vi "EDITORS_calculate_next_pos_for_keyboard_events.vi"(7 "direction":T1, 9 "SQL_rows":i32, 10 "editable_columns":i32[](array[numeric]), 11 "reference":refnum<vi>) -> ()   [LabVIEW 2019]
uses:
  _misc/directions.ctl
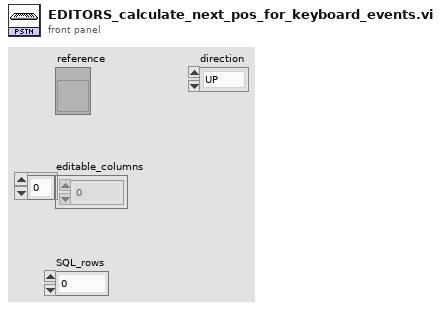
[diagram p1: front panel]
types:
  T1 = typedef "directions.ctl" = enum16{"UP", "DOWN", "LEFT", "RIGHT"}
  T2 = typedef "LVRowAndColumnTypeDef.ctl" = cluster{"Row":i32, "Column":i32}
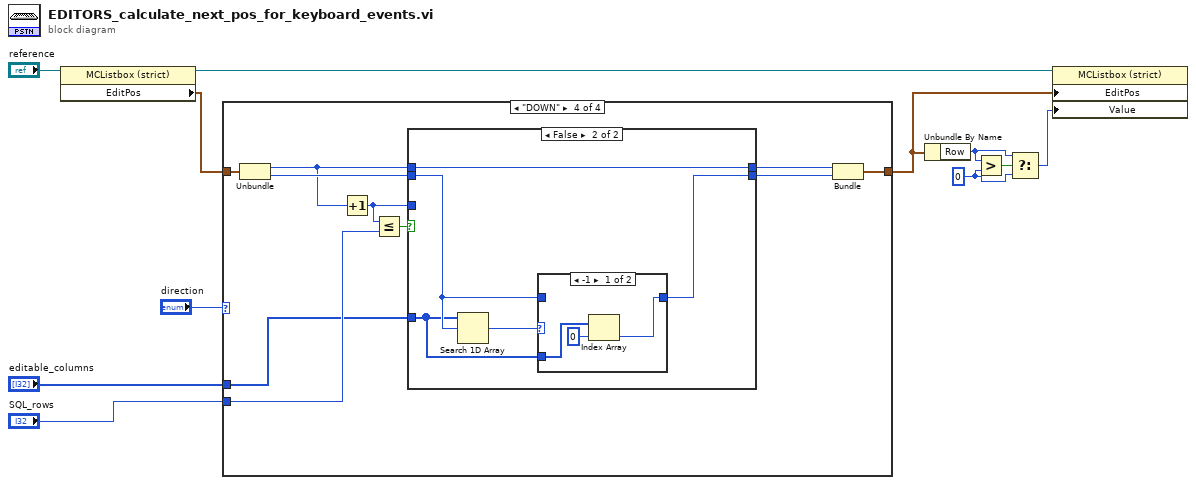
[diagram p0: block diagram]
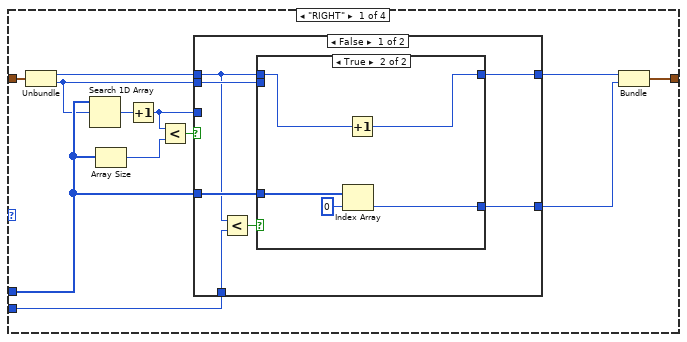
[diagram p2: hidden frame]
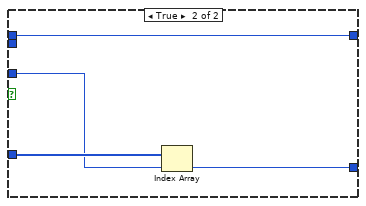
[diagram p4: hidden frame]
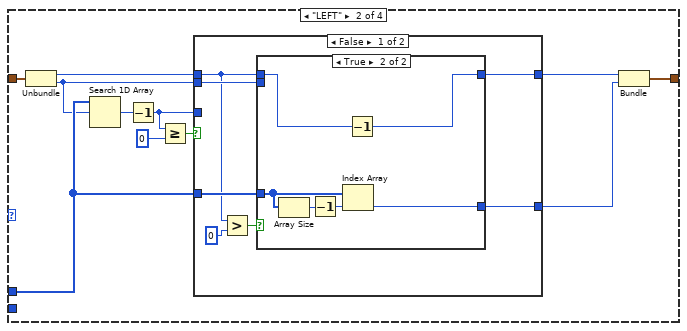
[diagram p5: hidden frame]
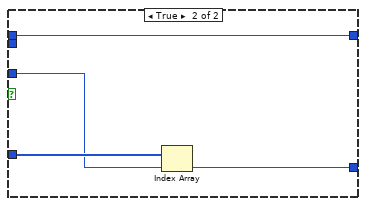
[diagram p7: hidden frame]
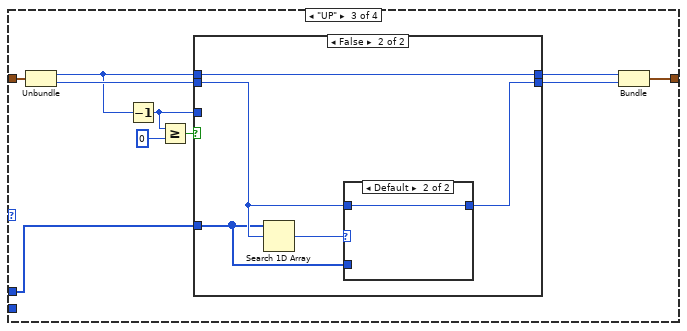
[diagram p8: hidden frame]
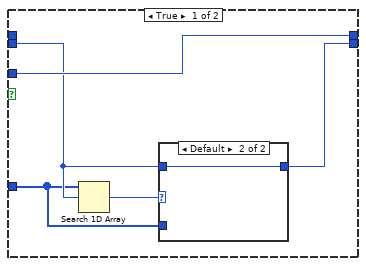
[diagram p9: hidden frame]
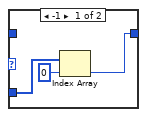
[diagram p10: hidden frame]
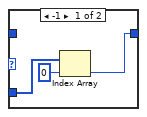
[diagram p11: hidden frame]
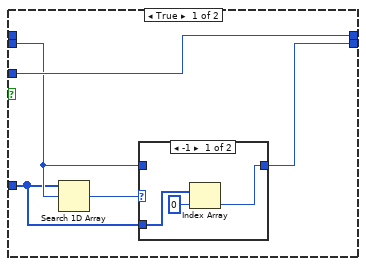
[diagram p12: hidden frame]
diagram:
  w2 = 0 ("lower limit")
  n1 = property on="Property Node" class="MCListbox (strict)"(reference="reference") -> (reference out=w10:refnum<vi>, "EditPos"=w11:T2)  [unwired: 1 in, 1 out]
  n2 = case shown="\"DOWN\"" "direction" {
    tunnel: w11 -> [w23 w52 w81 w109]
    tunnel: [w22 w51 w80 w108] -> w5
    tunnel: "editable_columns" -> [w18 w48 w72 w100]
    tunnel: "SQL_rows" -> [w12 _ _ w101]
    frame "RIGHT" {
      n3 = Unbundle(w23) -> ("Row"=w15:i32, "Column"=w13:i32)
      n4 = Search 1D Array(1D array=w18, element=w13) -> (index of element=w21:i32)  [unwired: 1 in]
      n5 = Array Size(array=w18) -> (size(s)=w20:i32)
      n6 = Increment(x=w21) -> (x+1=w17:i32)
      n7 = Less?(x=w17, y=w20) -> (x < y?=w19:bool)
      n8 = case shown="False" w19 {
        tunnel: w18 -> [w29 w41]
        tunnel: w17 -> [_ w40]
        tunnel: [w28 w39] -> w16
        tunnel: w15 -> [w25 w38]
        tunnel: [w30 w38] -> w14
        tunnel: w13 -> [w27 _]
        tunnel: w12 -> [w24 _]
        frame False {
          n9 = Less?(x=w25, y=w24) -> (x < y?=w26:bool)
          n10 = case shown="True" w26 {
            tunnel: w25 -> [w32 w37]
            tunnel: [w32 w36] -> w30
            tunnel: w29 -> [_ w34]
            tunnel: [w31 w35] -> w28
            tunnel: w27 -> [w31 _]
            frame False {
            }
            frame True {
              n11 = Index Array(array=w34, index=0) -> (element=w35:i32)
              n12 = Increment(x=w37) -> (x+1=w36:i32)
            }
          }
        }
        frame True {
          n13 = Index Array(array=w41, index=w40) -> (element=w39:i32)
        }
      }
      n14 = Bundle("Row"=w14, "Numeric"=w16) -> (w22:cluster{"Row":i32, "Numeric":i32})  [unwired: 1 in]
    }
    frame "LEFT" {
      n15 = Unbundle(w52) -> ("Row"=w45:i32, "Column"=w43:i32)
      n16 = Search 1D Array(1D array=w48, element=w43) -> (index of element=w50:i32)  [unwired: 1 in]
      n17 = Decrement(x=w50) -> (x-1=w47:i32)
      n18 = Greater Or Equal?(x=w47, y=0) -> (x >= y?=w49:bool)
      n19 = case shown="False" w49 {
        tunnel: w48 -> [w58 w71]
        tunnel: w47 -> [_ w70]
        tunnel: [w57 w69] -> w46
        tunnel: w45 -> [w54 w68]
        tunnel: [w59 w68] -> w44
        tunnel: w43 -> [w56 _]
        frame False {
          n20 = Greater?(x=w54, y=0) -> (0:w55:bool)
          n21 = case shown="True" w55 {
            tunnel: w54 -> [w61 w67]
            tunnel: [w61 w66] -> w59
            tunnel: w58 -> [_ w62]
            tunnel: [w60 w65] -> w57
            tunnel: w56 -> [w60 _]
            frame False {
            }
            frame True {
              n22 = Array Size(array=w62) -> (size(s)=w64:i32)
              n23 = Decrement(x=w64) -> (x-1=w63:i32)
              n24 = Index Array(array=w62, index=w63) -> (element=w65:i32)
              n25 = Decrement(x=w67) -> (x-1=w66:i32)
            }
          }
        }
        frame True {
          n26 = Index Array(array=w71, index=w70) -> (element=w69:i32)
        }
      }
      n27 = Bundle("Row"=w44, "Numeric"=w46) -> (w51:cluster{"Row":i32, "Numeric":i32})  [unwired: 1 in]
    }
    frame "UP" {
      n28 = Unbundle(w81) -> ("Row"=w74:i32, "Column"=w76:i32)
      n29 = Decrement(x=w74) -> (x-1=w78:i32)
      n30 = Greater Or Equal?(x=w78, y=0) -> (x >= y?=w79:bool)
      n31 = case shown="False" w79 {
        tunnel: w78 -> [w86 _]
        tunnel: w74 -> [_ w91]
        tunnel: [w86 w91] -> w77
        tunnel: w76 -> [w84 w94]
        tunnel: [w82 w92] -> w73
        tunnel: w72 -> [w83 w93]
        frame True {
          n32 = Search 1D Array(1D array=w83, element=w84) -> (index of element=w85:i32)  [unwired: 1 in]
          n33 = case shown="Default" w85 {
            tunnel: w84 -> [_ w90]
            tunnel: [w87 w90] -> w82
            tunnel: w83 -> [w89 _]
            frame -1 {
              n34 = Index Array(array=w89, index=0) -> (element=w87:i32)
            }
            frame Default {
            }
          }
        }
        frame False {
          n35 = Search 1D Array(1D array=w93, element=w94) -> (index of element=w95:i32)  [unwired: 1 in]
          n36 = case shown="Default" w95 {
            tunnel: w94 -> [_ w99]
            tunnel: [w96 w99] -> w92
            tunnel: w93 -> [w98 _]
            frame -1 {
              n37 = Index Array(array=w98, index=0) -> (element=w96:i32)
            }
            frame Default {
            }
          }
        }
      }
      n38 = Bundle("Row"=w77, "Column"=w73) -> (w80:cluster{"Row":i32, "Column":i32})  [unwired: 1 in]
    }
    frame "DOWN" {
      n39 = Unbundle(w109) -> ("Row"=w103:i32, "Column"=w104:i32)
      n40 = Increment(x=w103) -> (x+1=w106:i32)
      n41 = Less Or Equal?(x=w106, y=w101) -> (x <= y?=w107:bool)
      n42 = case shown="False" w107 {
        tunnel: w106 -> [w114 _]
        tunnel: w103 -> [_ w119]
        tunnel: [w114 w119] -> w105
        tunnel: w104 -> [w112 w122]
        tunnel: [w111 w121] -> w102
        tunnel: w100 -> [w110 w120]
        frame True {
          n43 = Search 1D Array(1D array=w110, element=w112) -> (index of element=w113:i32)  [unwired: 1 in]
          n44 = case shown="-1" w113 {
            tunnel: w112 -> [_ w118]
            tunnel: [w115 w118] -> w111
            tunnel: w110 -> [w117 _]
            frame -1 {
              n45 = Index Array(array=w117, index=0) -> (element=w115:i32)
            }
            frame Default {
            }
          }
        }
        frame False {
          n46 = Search 1D Array(1D array=w120, element=w122) -> (index of element=w123:i32)  [unwired: 1 in]
          n47 = case shown="-1" w123 {
            tunnel: w122 -> [_ w127]
            tunnel: [w124 w127] -> w121
            tunnel: w120 -> [w126 _]
            frame -1 {
              n48 = Index Array(array=w126, index=0) -> (element=w124:i32)
            }
            frame Default {
            }
          }
        }
      }
      n49 = Bundle("Row"=w105, "Column"=w102) -> (w108:cluster{"Row":i32, "Column":i32})  [unwired: 1 in]
    }
  }
  n50 = Unbundle By Name(w5) -> ("Row"=w3:i32)
  n51 = Greater?(x=w3, y=w2) -> (0:w4:bool)
  n52 = Select(t=w3, s=w4, f=w2) -> (s? t:f=w1:i32)
  n53 = property on="Property Node" class="MCListbox (strict)"(reference=w10, "EditPos"=w5, "Value"=w1) -> ()  [unwired: 1 in, 2 out]
